vi "ma_sml_Cascaded Decimation Filter (complex input) (No State).vi"(6 "reset?":bool, 7 "sml_Cascaded Decimation Filter (complex input) state in":T1={"unprocessed data state"=[], "final conditions state"=[], "sml_M-1 Decimator with IC (complex input) state"={"coefficients in reverse order state"=[], "max index for coefficients state"=1}} {"sml_M-1 Decimator with IC (complex input) state"."coefficients in reverse order state" format="%.2f"}, 10 "filter specification":cluster{"h":dbl[], "M":i32, "N":i32}={"h"=[5.017842402298822e-06, -3.6347034460970388e-06, -1.3387466661726196e-05, -7.845024922393745e-07, 2.4426233326325416e-05, 1.069359798524219e-05, -3.953063749330246e-05, -3.449004233474014e-05, 5.166753079423074e-05, 7.580241145008019e-05, -5.202393998060288e-05, -0.00013695088647737978, 2.644152675547298e-05, 0.00021368550203212212, 4.161120271313457e-05, -0.00029287162186333453, -0.00016800576540118464, 0.0003500423446652448, 0.0003622558258869545, -0.0003494082460775069, -0.0006207716924522643, 0.0002469255850065727, 0.0009198920769782536, 2.737152974592998e-06, -0.0012106430242707475, -0.0004354608386366535, 0.0014171861215696209, 0.0010641089924028914, -0.0014408790456388381, -0.0018642019842870067, 0.0011711992096026893, 0.0027616563661223034, -0.0005036324432956759, -0.0036258957001366787, -0.0006367796558850806, 0.00427135221964554, 0.0022690471070142635, -0.00446945340095769, -0.004330934234499924, 0.00397160860790426, 0.006659262862425487, -0.0025415780984074064, -0.008979784594616836, -6.458801396183972e-06, 0.010908888620151816, 0.0037696314078308054, -0.011966313250411517, -0.008724382417252324, 0.01159298865991561, 0.01470707822463853, -0.009159906105557362, -0.021412246936221454, 0.003936970653343424, 0.02841100284536082, 0.005054265927768018, -0.035189042115008715, -0.01953602497219576, 0.0412002318343485, 0.043765506251261, -0.04592888866554608, -0.09358505861942605, 0.048951961493948204, 0.3140370477958766, 0.45000812179125654, 0.3140370477958766, 0.048951961493948204, -0.09358505861942605, -0.04592888866554608, 0.043765506251261, 0.0412002318343485, -0.01953602497219576, -0.035189042115008715, 0.005054265927768018, 0.02841100284536082, 0.003936970653343424, -0.021412246936221454, -0.009159906105557362, 0.01470707822463853, 0.01159298865991561, -0.008724382417252324, -0.011966313250411517, 0.0037696314078308054, 0.010908888620151816, -6.458801396183972e-06, -0.008979784594616836, -0.0025415780984074064, 0.006659262862425487, 0.00397160860790426, -0.004330934234499924, -0.00446945340095769, 0.0022690471070142635, 0.00427135221964554, -0.0006367796558850806, -0.0036258957001366787, -0.0005036324432956759, 0.0027616563661223034, 0.0011711992096026893, -0.0018642019842870067, -0.0014408790456388381, 0.0010641089924028914, 0.0014171861215696209, -0.0004354608386366535, -0.0012106430242707475, 2.737152974592998e-06, 0.0009198920769782536, 0.0002469255850065727, -0.0006207716924522643, -0.0003494082460775069, 0.0003622558258869545, 0.0003500423446652448, -0.00016800576540118464, -0.00029287162186333453, 4.161120271313457e-05, 0.00021368550203212212, 2.644152675547298e-05, -0.00013695088647737978, -5.202393998060288e-05, 7.580241145008019e-05, 5.166753079423074e-05, -3.449004233474014e-05, -3.953063749330246e-05, 1.069359798524219e-05, 2.4426233326325416e-05, -7.845024922393745e-07, -1.3387466661726196e-05, -3.6347034460970388e-06, 5.017842402298822e-06], "M"=2, "N"=0} {"h" format="%.2f"}, 11 "x":cdb[](array[numeric]) format="%.2f") -> (3 "y":cdb[](array[numeric]) format="%.2f", 5 "sml_Cascaded Decimation Filter (complex input) state out":T1={"unprocessed data state"=[], "final conditions state"=[], "sml_M-1 Decimator with IC (complex input) state"={"coefficients in reverse order state"=[], "max index for coefficients state"=1}} {"sml_M-1 Decimator with IC (complex input) state"."coefficients in reverse order state" format="%.2f"})   [LabVIEW 2020, in "NI_MAPro.lvlib"]
doc: "This function filters input signal x and then decimates the output by M^N. It is equal to N stage of decimation by M filter. Each of the decimation by M filter has the same filter coefficients."
uses:
  NI_MAPro.lvlib
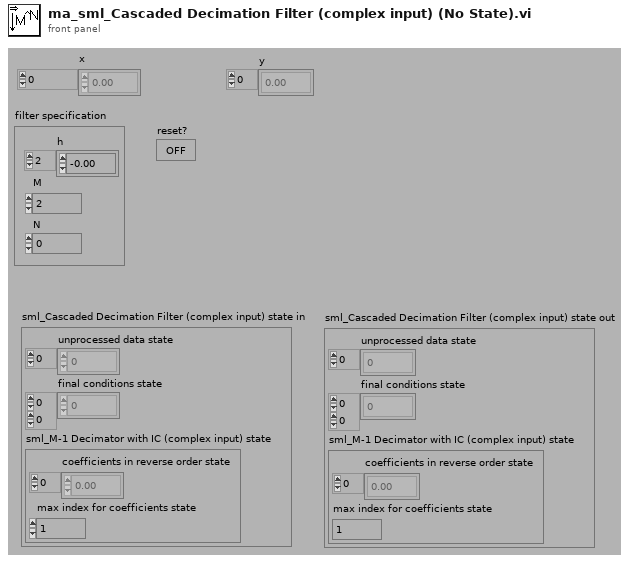
[diagram p1: front panel]
types:
  T1 = cluster{"unprocessed data state":cdb[], "final conditions state":cdb[][], "sml_M-1 Decimator with IC (complex input) state":cluster{"coefficients in reverse order state":dbl[], "max index for coefficients state":i32}}
  T2 = cluster{"coefficients in reverse order state":dbl[], "max index for coefficients state":i32}
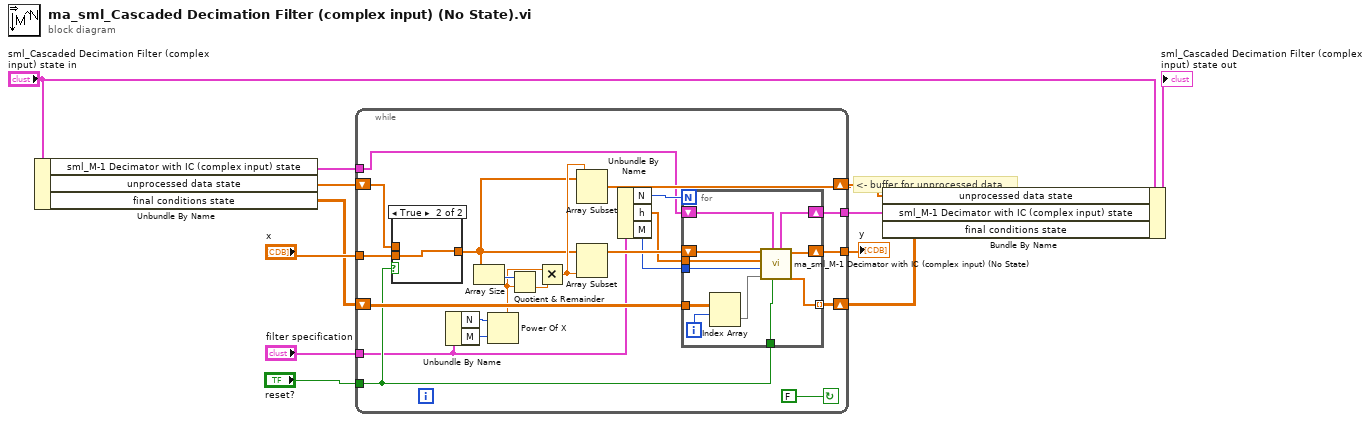
[diagram p0: block diagram]
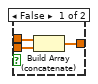
[diagram p2: hidden frame]
diagram:
  # "<- buffer for unprocessed data"
  n1 = Unbundle By Name("sml_Cascaded Decimation Filter (complex input) state in") -> ("sml_M-1 Decimator with IC (complex input) state"=w5:T2, "unprocessed data state"=w7:cdb[], "final conditions state"=w6:cdb[][])
  n2 = while {
    tunnel: "filter specification" -> [w15]
    tunnel: "reset?" -> [w17]
    tunnel: [w19] -> w11
    tunnel: "x" -> [w31]
    shift-left: w7 -> [w32]
    shift-right: [w18] -> w3
    shift-left: w6 -> [w33]
    shift-right: [w34] -> w4
    tunnel: w5 -> [w14]
    tunnel: [w13] -> w2
    stop <- FALSE continue-if-true
    n3 = case shown="True" w17 {
      tunnel: w32 -> [w37 _]
      tunnel: w31 -> [w36 w38]
      tunnel: [w35 w38] -> w25
      frame False {
        n4 = Build Array (concatenate)(w37, w36) -> (w35:cdb[])
      }
      frame True {
      }
    }
    n5 = Unbundle By Name(w15) -> ("N"=w29:i32, "M"=w28:i32)
    n6 = Array Size(array=w25) -> (size(s)=w30:i32)
    n7 = Power Of X(1:w28, 2:w29) -> (0:w20:dbl)
    n8 = Quotient & Remainder(x=w30, y=w20) -> (floor(x/y)=w21:dbl)  [unwired: 1 out]
    n9 = Multiply(x=w20, y=w21) -> (x*y=w26:dbl)
    n10 = Array Subset(array=w25, index=w26) -> (w18:cdb[])  [unwired: 1 in]
    n11 = Array Subset(array=w25, length=w26) -> (w27:cdb[])  [unwired: 1 in]
    n12 = Unbundle By Name(w15) -> ("N"=w24:i32, "h"=w22:dbl[], "M"=w23:i32)
    n13 = for {
      N: w24 -> [_]
      tunnel: [w49] -> w34 mode=indexing
      tunnel: w33 -> [w43]
      tunnel: w23 -> [w48]
      shift-right: [w46] -> w19
      shift-left: w27 -> [w47]
      tunnel: w22 -> [w42]
      tunnel: w17 -> [w41]
      shift-right: [w39] -> w13
      shift-left: w14 -> [w40]
      i -> [w44]
      n14 = Index Array(array=w43, index (row)=w44) -> (element=w45:cdb[])  [unwired: 1 in]
      n15 = call "ma_sml_M-1 Decimator with IC (complex input) (No State).vi"("reset?"=w41, "sml_M-1 Decimator with IC (complex input) state in"=w40, "initial conditions"=w45, "M"=w48, "coefficients"=w42, "x"=w47) -> ("y"=w46:cdb[], "final conditions"=w49:cdb[], "sml_M-1 Decimator with IC (complex input) state out"=w39:T2)  [unwired: 3 out]
    }
  }
  "y" <- w11
  n16 = Bundle By Name(cluster="sml_Cascaded Decimation Filter (complex input) state in", "unprocessed data state"=w3, "sml_M-1 Decimator with IC (complex input) state"=w2, "final conditions state"=w4) -> (→"sml_Cascaded Decimation Filter (complex input) state out":T1)
